vi "BlackImageTest.vi"() -> ()   [LabVIEW 2013]
panel:
  out "Black?":bool
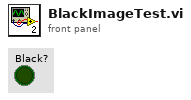
[diagram p1: front panel]
types:
  T1 = typedef "Image Type" = u32
  T2 = typedef "IMAQ Image.ctl" = refnum<image>
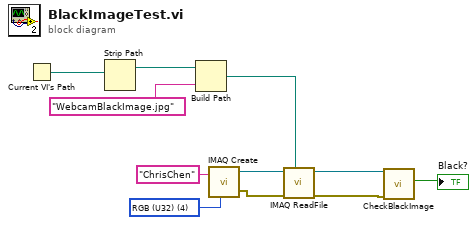
[diagram p0: block diagram]
diagram:
  w4 = T1 4 items=["Grayscale (U8)", "Grayscale (I16)", "Grayscale (SGL)", "Complex (CSG)", "RGB (U32)", "HSL (U32)", "RGB (U64)", "Grayscale (U16)"] ("Image Type")
  n1 = Current VI's Path() -> (path=w8:path)
  n2 = Strip Path(path=w8) -> (stripped path=w7:path)  [unwired: 1 out]
  n3 = Build Path(base path=w7, name or relative path="WebcamBlackImage.jpg") -> (appended path=w5:path)
  n4 = call "IMAQ Create"("Image Name"="ChrisChen", "Image Type"=w4) -> ("New Image"=w11:T2, "error out"=w10:errorcluster)  [unwired: 3 in]
  n5 = call "IMAQ ReadFile"("File Path"=w5, "error in (no error)"=w10, "Image"=w11) -> ("error out"=w2:errorcluster, "Image Out"=w3:T2)  [unwired: 4 in, 3 out]
  n6 = call "CheckBlackImage.vi"("error in"=w2, "Image In"=w3) -> ("Black?"=→"Black?":bool)  [unwired: 7 in, 2 out]
